vi "Session Initialization Details from Resource Name.vi"(11 "resource name":string) -> (3 "session initialization details":T1)   [LabVIEW 2020, in "MeasurementServerTests.lvlib"]
uses:
  MeasurementServerTests.lvlib
  Runtime/MeasurementLink Instrument/IInstrument/Session Initialization Details.ctl
  Runtime/MeasurementLink Instrument/IInstrument/IInstrument.lvclass
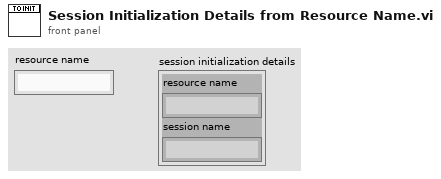
[diagram p1: front panel]
types:
  T1 = typedef "MeasurementLink Instrument.lvlib/IInstrument.lvclass/Session Initialization Details.ctl" = cluster{"resource name":string, "session name":string}
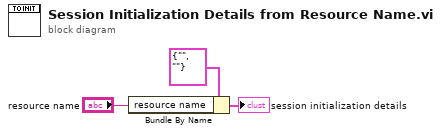
[diagram p0: block diagram]
diagram:
  n1 = Bundle By Name(cluster=T1 {"resource name"="", "session name"=""} ("session initialization details"), "resource name"="resource name") -> (→"session initialization details":T1)
